vi "GetLatestTimes.vi"(8 "error in (no error)":errorcluster, 11 "FAMM in":refnum<class "FAMM.lvclass">) -> (0 "error out":errorcluster, 1 "AverTimes":timestamp[](array[timestamp]), 2 "LatestTimes":timestamp[](array[timestamp]), 3 "FAMM out":refnum<class "FAMM.lvclass">)   [LabVIEW 2014, in "FAMM.lvclass"]
doc: "Get the latest times from all the PAQ resolution layers the FAMM buffer"
uses:
  FAMM.lvclass
  Common/controls/GlobalClassRefs.vi
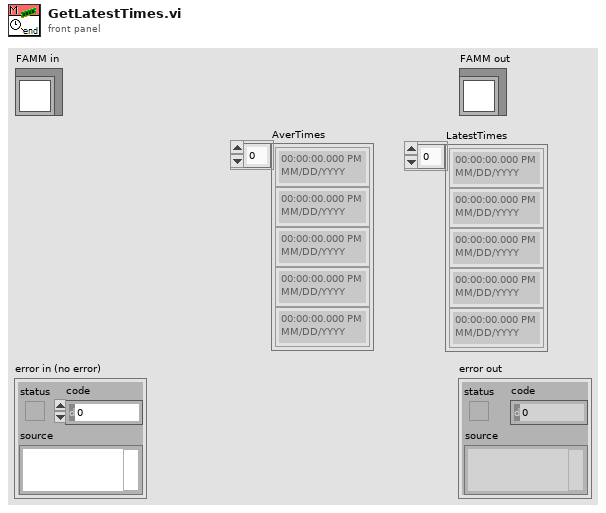
[diagram p1: front panel]
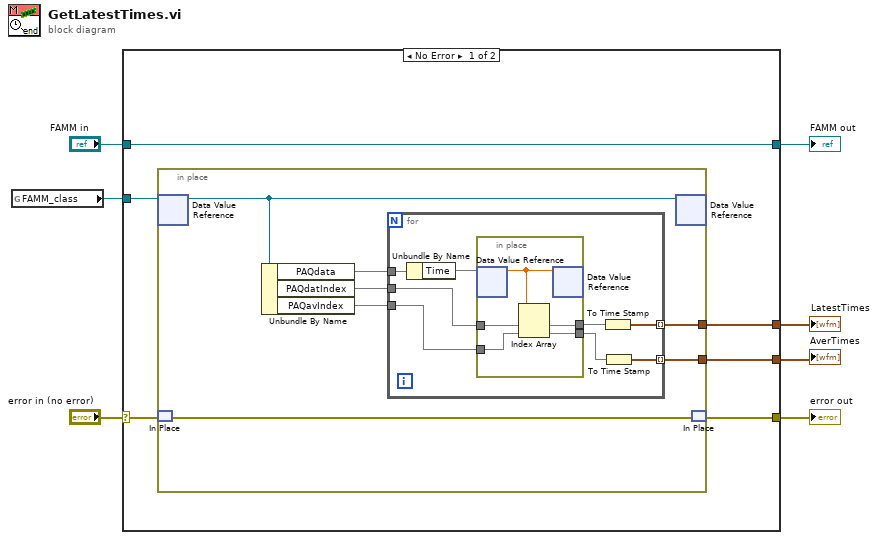
[diagram p0: block diagram]
diagram:
  n1 = global read "GlobalClassRefs.vi" "FAMM_class"() -> (w1:refnum<data-value>)
  n2 = case shown="No Error" "error in (no error)" {
    selector: "error in (no error)" -> [w13 w35]
    tunnel: [w10 w35] -> w6
    tunnel: [w12 w34] -> w4
    tunnel: "FAMM in" -> [w12 w34]
    tunnel: w1 -> [w11 _]
    tunnel: [w9 _] -> w3
    tunnel: [w8 _] -> w2
    frame No Error {
      n3 = in-place {
        in-place-border: [w18] -> w9
        in-place-border: [w14] -> w8
        n4 = in-place-dvr #1(w11) -> (w20:refnum<class "FAMM.lvclass">)  [unwired: 1 out]
        n5 = in-place-match #2(w13) -> (w19:errorcluster)
        n6 = Unbundle By Name(w20) -> ("PAQdata"=w17, "PAQdatIndex"=w16, "PAQavIndex"=w15)
        n7 = for {
          tunnel: w17 -> [w28]
          tunnel: w16 -> [w26]
          tunnel: [w24] -> w18 mode=indexing
          tunnel: w15 -> [w23]
          tunnel: [w21] -> w14 mode=indexing
          n8 = Unbundle By Name(w28) -> ("Time"=w27)
          n9 = in-place {
            in-place-border: w26 -> [w32]
            in-place-border: [w31] -> w25
            in-place-border: w23 -> [w30]
            in-place-border: [w29] -> w22
            n10 = in-place-dvr #3(w27) -> (w33:dbl)  [unwired: 1 out]
            n11 = Index Array(array=w33, index #1=w32, index #2=w30) -> (element #1=w31, element #2=w29)
            n12 = in-place-dvr #3(w33) -> ()  [unwired: 2 out]
          }
          n13 = To Time Stamp(1:w25) -> (0:w24:timestamp)
          n14 = To Time Stamp(1:w22) -> (0:w21:timestamp)
        }
        n15 = in-place-dvr #1(w20) -> ()  [unwired: 2 out]
        n16 = in-place-match #2(w19) -> (w10:errorcluster)
      }
    }
    frame Error {
    }
  }
  "error out" <- w6
  "FAMM out" <- w4
  "LatestTimes" <- w3
  "AverTimes" <- w2
